vi "10.RectangleMove.vi"   [LabVIEW 2017]
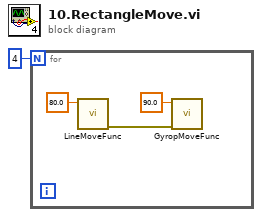
[diagram p0: block diagram]
diagram:
  n1 = for {
    N: 4 -> [_]
    n2 = call "LineMoveFunc.vi"("小车期望运\n行的距离"=80.0 ("小车期望运\n行的距离")) -> ("error out"=w3:errorcluster)  [unwired: 10 in]
    n3 = call "GyropMoveFunc.vi"("error in (no error)"=w3, "期望旋转角度"=90.0) -> ()  [unwired: 9 in, 1 out]
  }
